vi "UDP_comm_state_machine.vi"(6 "Data to send":T1, 8 "error in (no error)":errorcluster, 9 "UDP State":T4, 11 "UDP Pproperties":T3={"Remote Host Port"=9999, "Remote Host IP"="127.0.0.1", "write_ID"=enum."0"}) -> (0 "error out":errorcluster, 1 "error code":i32, 3 "Data to read OUT":T2)   [LabVIEW 2012]
uses:
  UDP_state.ctl
  DataToSend.ctl
panel:
  out "error IO":errorcluster
  out "offset past number":i32
  out "substring":string
  out "number":dbl
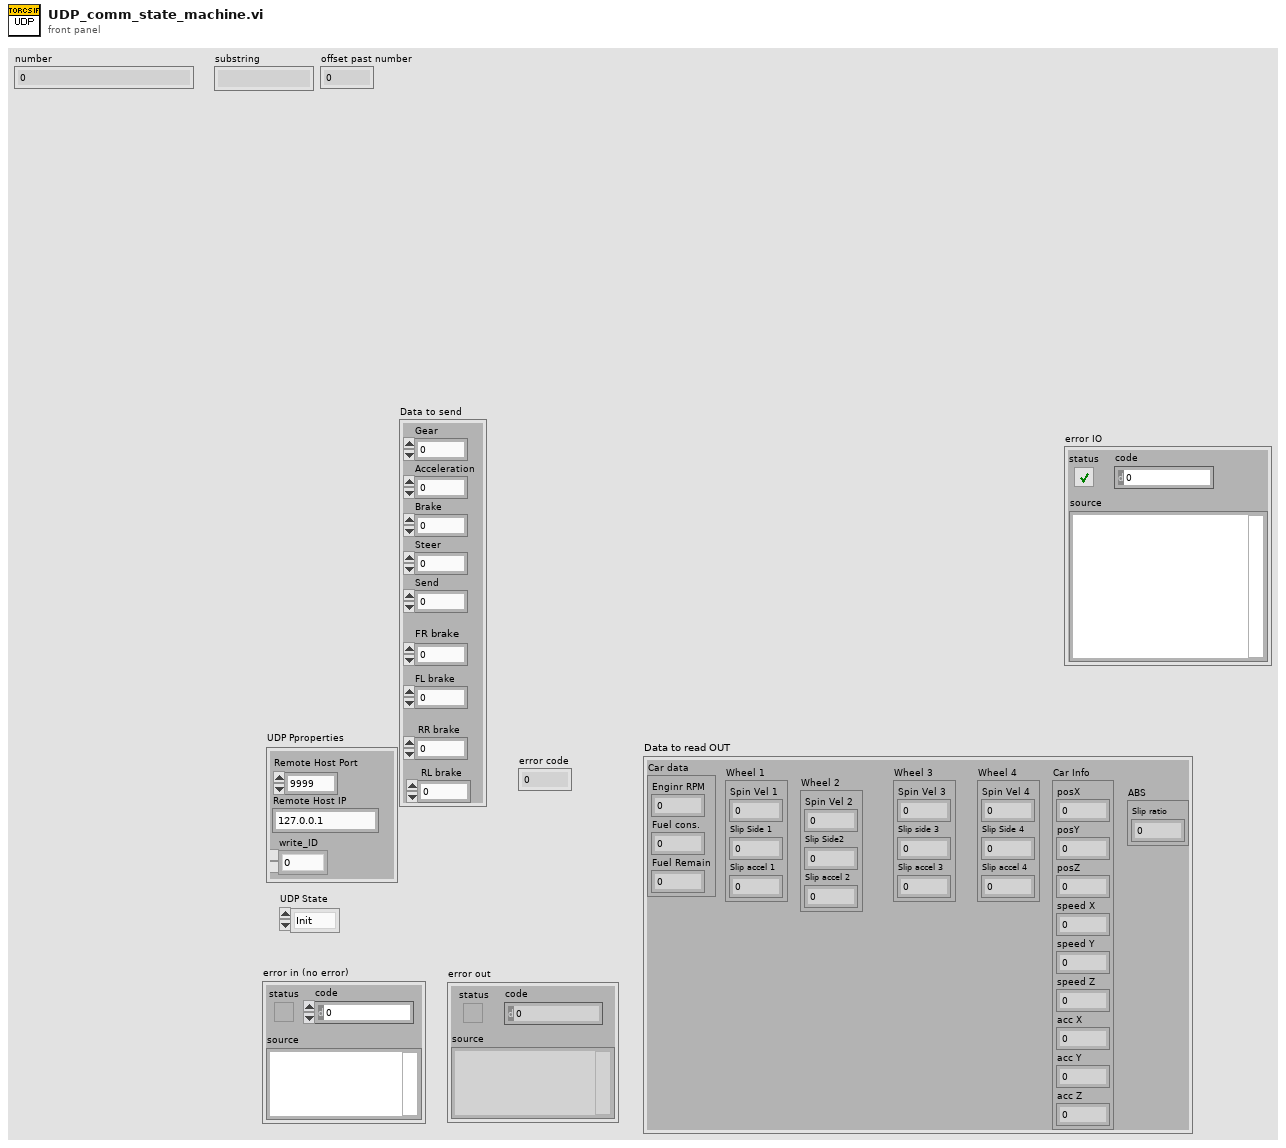
[diagram p1: front panel]
types:
  T1 = typedef "DataToSend.ctl" = cluster{"Gear":dbl, "Acceleration":dbl, "Brake":dbl, "Steer":dbl, "Send":dbl, "FR brake":dbl, "FL brake":dbl, " RR brake":dbl, " RL brake":dbl}
  T2 = cluster{"Car data ":cluster{"Enginr RPM":dbl, "Fuel cons.":dbl, "Fuel Remain":dbl}, "Wheel 1":cluster{"Spin Vel 1":dbl, "Slip Side 1":dbl, "Slip accel 1":dbl}, "Wheel 2":cluster{"Spin Vel 2":dbl, "Slip Side2":dbl, "Slip accel 2":dbl}, "Wheel 3":cluster{"Spin Vel 3":dbl, "Slip side 3":dbl, "Slip accel 3":dbl}, "Wheel 4":cluster{"Spin Vel 4":dbl, "Slip Side 4":dbl, "Slip accel 4":dbl}, "Car Info":cluster{"posX":dbl, "posY":dbl, "posZ":dbl, "speed X":dbl, "speed Y":dbl, "speed Z":dbl, "acc X":dbl, "acc Y":dbl, "acc Z":dbl}, "ABS":cluster{"Slip ratio":dbl}}
  T3 = cluster{"Remote Host Port":u16, "Remote Host IP":string, "write_ID":enum32{"0", "1", "2", "3", "4"}}
  T4 = typedef "UDP_state.ctl" = enum16{"Init", "Write", "Read", "Close"}
  T5 = cluster{"Enginr RPM":dbl, "Fuel cons.":dbl, "Fuel Remain":dbl}
  T6 = cluster{"posX":dbl, "posY":dbl, "posZ":dbl, "speed X":dbl, "speed Y":dbl, "speed Z":dbl, "acc X":dbl, "acc Y":dbl, "acc Z":dbl}
  T7 = cluster{"Spin Vel 1":dbl, "Slip Side 1":dbl, "Slip accel 1":dbl}
  T8 = cluster{"Spin Vel 2":dbl, "Slip Side2":dbl, "Slip accel 2":dbl}
  T9 = cluster{"Spin Vel 3":dbl, "Slip side 3":dbl, "Slip accel 3":dbl}
  T10 = cluster{"Spin Vel 4":dbl, "Slip Side 4":dbl, "Slip accel 4":dbl}
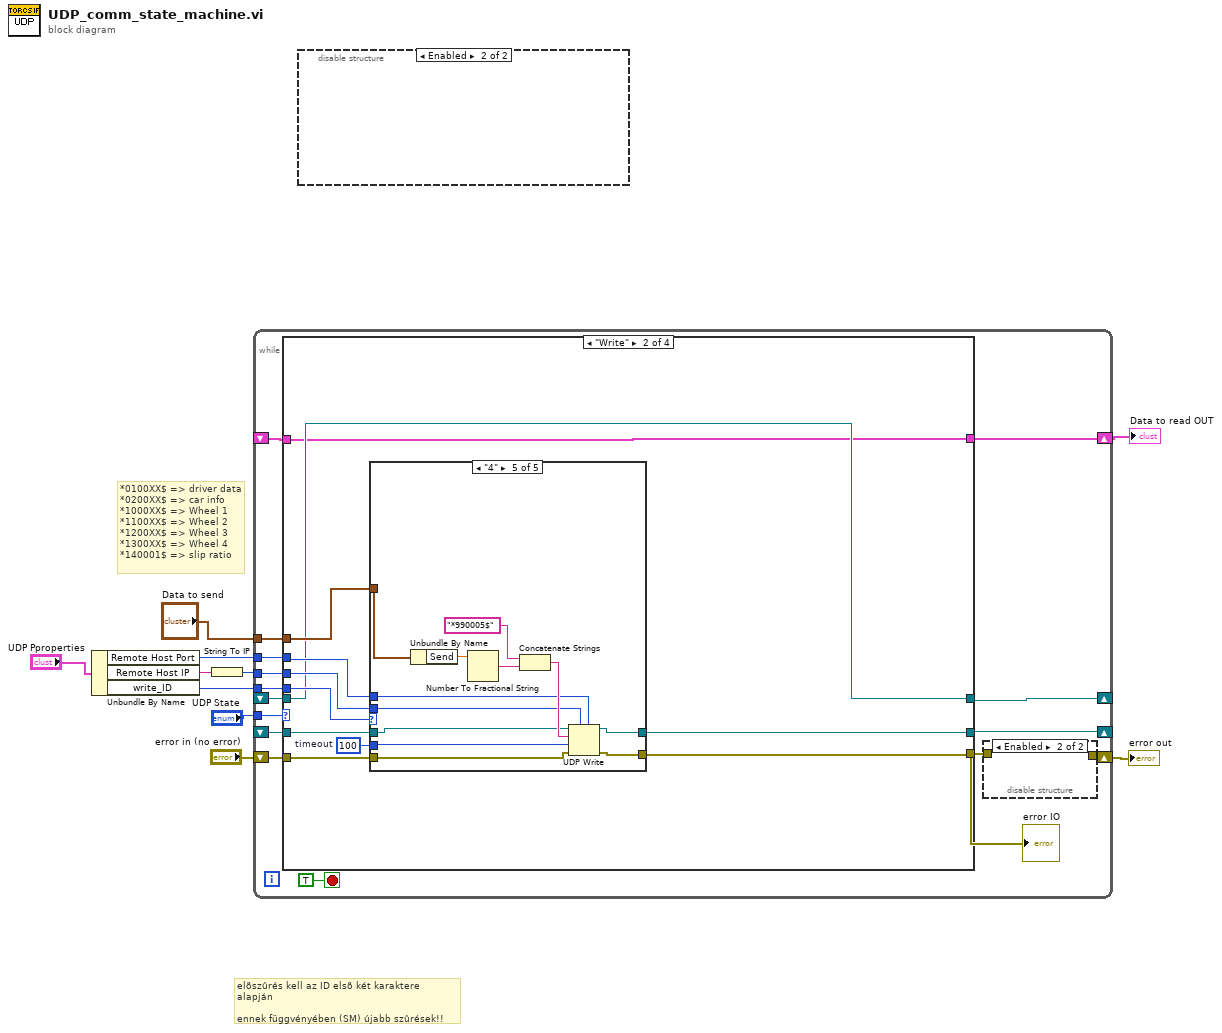
[diagram p0: block diagram]
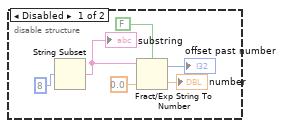
[diagram p2: hidden frame]
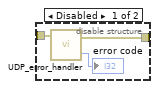
[diagram p3: hidden frame]
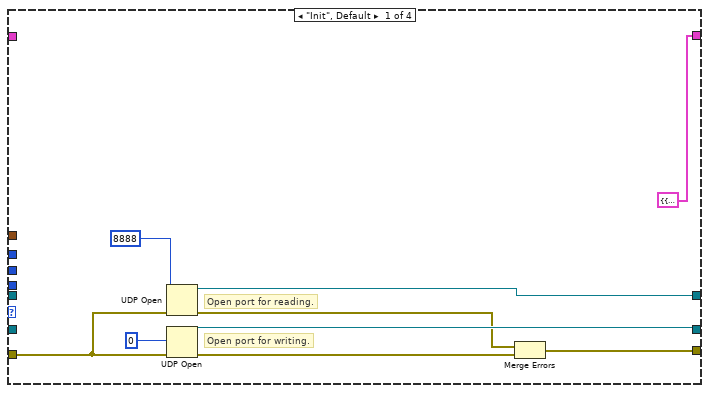
[diagram p4: hidden frame]
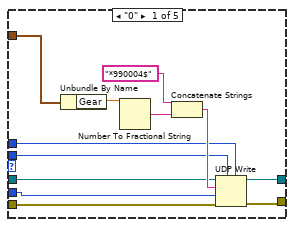
[diagram p5: hidden frame]
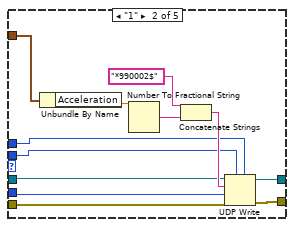
[diagram p6: hidden frame]
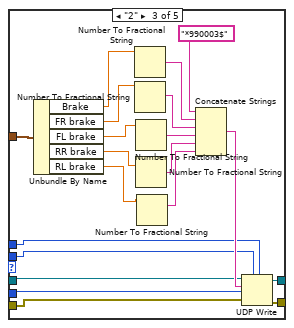
[diagram p7: hidden frame]
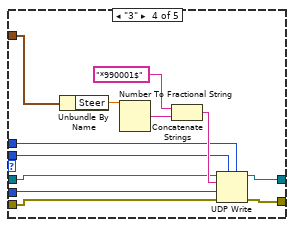
[diagram p8: hidden frame]
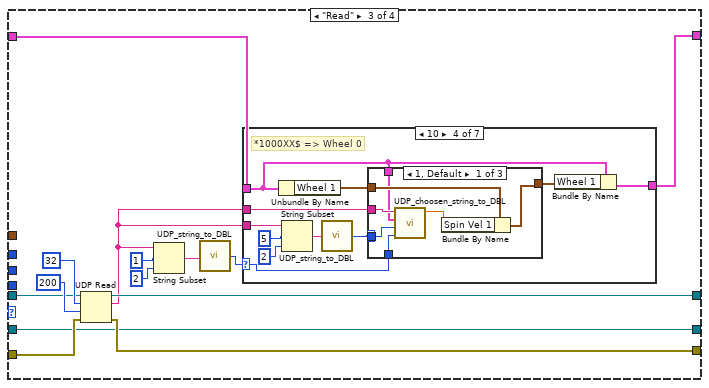
[diagram p9: hidden frame]
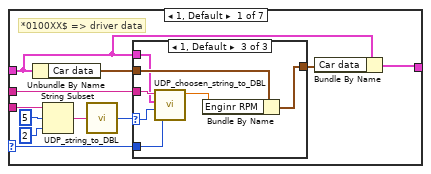
[diagram p10: hidden frame]
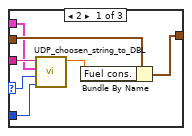
[diagram p11: hidden frame]
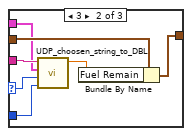
[diagram p12: hidden frame]
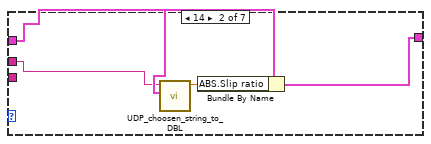
[diagram p13: hidden frame]
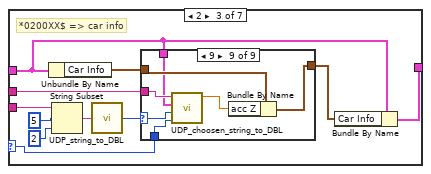
[diagram p14: hidden frame]
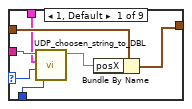
[diagram p15: hidden frame]
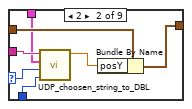
[diagram p16: hidden frame]
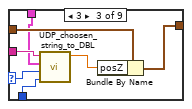
[diagram p17: hidden frame]
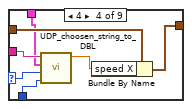
[diagram p18: hidden frame]
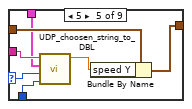
[diagram p19: hidden frame]
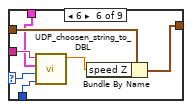
[diagram p20: hidden frame]
diagram:
  # "elõszûrés kell az ID elsõ két karaktere alapján\n\nennek függvényében (SM) újabb szûrések!!"
  # "*0100XX$ => driver data\n*0200XX$ => car info\n*1000XX$ => Wheel 1\n*1100XX$ => Wheel 2\n*1200XX$ => Wheel 3\n*1300XX$ => Wheel 4\n*140001$ => slip ratio"
  n1 = Unbundle By Name("UDP Pproperties") -> ("Remote Host Port"=w5:u16, "Remote Host IP"=w4:string, "write_ID"=w3:enum32{"0", "1", "2", "3", "4"})
  n2 = String To IP(1:w4) -> (0:w9:u32)
  n3 = while {
    shift-right: [w24] -> _
    shift-left: _ -> [w23]
    shift-right: [w13] -> w10
    shift-left: "error in (no error)" -> [w21]
    tunnel: "Data to send" -> [w22]
    shift-right: [w12] -> w2
    shift-left: _ -> [w11]
    tunnel: w5 -> [w20]
    tunnel: w9 -> [w19]
    tunnel: "UDP State" -> [w18]
    tunnel: w3 -> [w17]
    shift-right: [w16] -> _
    shift-left: _ -> [w15]
    stop <- TRUE stop-if-true
    n4 = case shown="\"Write\"" w18 {
      tunnel: [w37 w43 w124 w376] -> w24
      tunnel: w21 -> [w33 w47 w129 w374]
      tunnel: [w35 w42 w127 w372] -> w14
      tunnel: w23 -> [_ w48 w124 w377]
      tunnel: w22 -> [_ w46 _ _]
      tunnel: w11 -> [_ w39 w118 w369]
      tunnel: w20 -> [_ w45 _ _]
      tunnel: w19 -> [_ w44 _ _]
      tunnel: w17 -> [_ w41 _ _]
      tunnel: [w31 w40 w125 w370] -> w16
      tunnel: w15 -> [_ w40 w126 w375]
      tunnel: [T2 {"Car data "={"Enginr RPM"=0.0, "Fuel cons."=0.0, "Fuel Remain"=0.0}, "Wheel 1"={"Spin Vel 1"=0.0, "Slip Side 1"=0.0, "Slip accel 1"=0.0}, "Wheel 2"={"Spin Vel 2"=0.0, "Slip Side2"=0.0, "Slip accel 2"=0.0}, "Wheel 3"={"Spin Vel 3"=0.0, "Slip side 3"=0.0, "Slip accel 3"=0.0}, "Wheel 4"={"Spin Vel 4"=0.0, "Slip Side 4"=0.0, "Slip accel 4"=0.0}, "Car Info"={"posX"=0.0, "posY"=0.0, "posZ"=0.0, "speed X"=0.0, "speed Y"=0.0, "speed Z"=0.0, "acc X"=0.0, "acc Y"=0.0, "acc Z"=0.0}, "ABS"={"Slip ratio"=0.0}} ("Data to read OUT") w39 w119 w369] -> w12
      frame "Init", Default {
        # "Open port for writing."
        # "Open port for reading."
        n5 = UDP Open(8:w33, 11:u16 8888 ("port")) -> (port=w31:refnum<k16>, 0:w32:errorcluster)  [unwired: 3 in, 1 out]
        n6 = UDP Open(8:w33, 11:u16 0 ("port")) -> (port=w37:refnum<k16>, 0:w36:errorcluster)  [unwired: 3 in, 1 out]
        n7 = Merge Errors(w32, w36) -> (w35:errorcluster)
      }
      frame "Write" {
        w38 = 100  # timeout
        n8 = case shown="\"4\"" w41 {
          tunnel: w48 -> [w56 w63 w84 w97 w111]
          tunnel: w47 -> [w55 w61 w82 w96 w109]
          tunnel: w46 -> [w54 w66 w81 w100 w113]
          tunnel: w45 -> [w53 w65 w86 w98 w106]
          tunnel: w44 -> [w52 w64 w85 w99 w105]
          tunnel: [w51 w68 w87 w94 w107] -> w43
          tunnel: [w50 w67 w88 w93 w108] -> w42
          tunnel: w38 -> [w49 w62 w83 w95 w110]
          frame "0" {
            n9 = Unbundle By Name(w54) -> ("Gear"=w60:dbl)
            n10 = Number To Fractional String(number=w60) -> (F-format string=w59:string)  [unwired: 3 in]
            n11 = Concatenate Strings("*990004$", w59) -> (w58:string)
            n12 = UDP Write(address=w52, port or service name=w53, connection ID=w56, data in=w58, 8:w55, 9:w49) -> (error out=w50:errorcluster, 3:w51:refnum<k16>)
          }
          frame "1" {
            n13 = Unbundle By Name(w66) -> ("Acceleration"=w72:dbl)
            n14 = Number To Fractional String(number=w72) -> (F-format string=w71:string)  [unwired: 3 in]
            n15 = Concatenate Strings("*990002$", w71) -> (w69:string)
            n16 = UDP Write(address=w64, port or service name=w65, connection ID=w63, data in=w69, 8:w61, 9:w62) -> (error out=w67:errorcluster, 3:w68:refnum<k16>)
          }
          frame "2" {
            n17 = Unbundle By Name(w81) -> ("Brake"=w89:dbl, "FR brake"=w80:dbl, "FL brake"=w79:dbl, "RR brake"=w78:dbl, "RL brake"=w77:dbl)
            n18 = Number To Fractional String(number=w89) -> (F-format string=w91:string)  [unwired: 3 in]
            n19 = Number To Fractional String(number=w80) -> (F-format string=w76:string)  [unwired: 3 in]
            n20 = Number To Fractional String(number=w79) -> (F-format string=w75:string)  [unwired: 3 in]
            n21 = Number To Fractional String(number=w78) -> (F-format string=w74:string)  [unwired: 3 in]
            n22 = Number To Fractional String(number=w77) -> (F-format string=w73:string)  [unwired: 3 in]
            n23 = Concatenate Strings("*990003$", w91, w76, w75, w74, w73) -> (w92:string)
            n24 = UDP Write(address=w85, port or service name=w86, connection ID=w84, data in=w92, 8:w82, 9:w83) -> (error out=w88:errorcluster, 3:w87:refnum<k16>)
          }
          frame "3" {
            n25 = Unbundle By Name(w100) -> ("Steer"=w101:dbl)
            n26 = Number To Fractional String(number=w101) -> (F-format string=w103:string)  [unwired: 3 in]
            n27 = Concatenate Strings("*990001$", w103) -> (w102:string)
            n28 = UDP Write(address=w99, port or service name=w98, connection ID=w97, data in=w102, 8:w96, 9:w95) -> (error out=w93:errorcluster, 3:w94:refnum<k16>)
          }
          frame "4" {
            n29 = Unbundle By Name(w113) -> ("Send"=w112:dbl)
            n30 = Number To Fractional String(number=w112) -> (F-format string=w115:string)  [unwired: 3 in]
            n31 = Concatenate Strings("*990005$", w115) -> (w116:string)
            n32 = UDP Write(address=w105, port or service name=w106, connection ID=w111, data in=w116, 8:w109, 9:w110) -> (error out=w108:errorcluster, 3:w107:refnum<k16>)
          }
        }
      }
      frame "Read" {
        n33 = UDP Read(connection ID=w126, max size (548)=32, timeout ms (25000)=200, 8:w129) -> (data out=w117:string, error out=w127:errorcluster, 3:w125:refnum<k16>)  [unwired: 2 out]
        n34 = String Subset(string=w117, offset (0)=1, length (rest)=2 ("length (rest)")) -> (substring=w121:string)
        n35 = call "UDP_string_to_DBL.vi"("input string"=w121) -> ("output number"=w120:i32)
        n36 = case shown="10" w120 {
          selector: w120 -> [w133 _ w168 w243 w275 w308 w338]
          tunnel: w118 -> [w131 w165 w167 w242 w276 w305 w337]
          tunnel: w117 -> [w139 _ w170 w248 w280 w312 w344]
          tunnel: w117 -> [w137 w164 w171 w246 w274 w306 w340]
          tunnel: [w132 w166 w172 w244 w279 w311 w343] -> w119
          frame 1, Default {
            # "*0100XX$ => driver data"
            n37 = Unbundle By Name(w131) -> ("Car data"=w138:T5)
            n38 = String Subset(string=w139, offset (0)=5, length (rest)=2 ("length (rest)")) -> (substring=w136:string)
            n39 = call "UDP_string_to_DBL.vi"("input string"=w136) -> ("output number"=w134:i32)
            n40 = case shown="1, Default" w134 {
              selector: w134 -> [w144 w151 w158]
              tunnel: w138 -> [w147 w154 w162]
              tunnel: w137 -> [w145 w152 w159]
              tunnel: [w146 w153 w160] -> w135
              tunnel: w133 -> [w143 w150 w157]
              tunnel: w131 -> [w142 w149 w156]
              frame 2 {
                n41 = call "UDP_choosen_string_to_DBL.vi"("main ID"=w143, "secondary ID"=w144, "Data to read"=w142, "input string"=w145) -> ("output number"=w148:dbl)  [unwired: 3 in]
                n42 = Bundle By Name(cluster=w147, "Fuel cons."=w148) -> (w146:T5)
              }
              frame 3 {
                n43 = call "UDP_choosen_string_to_DBL.vi"("main ID"=w150, "secondary ID"=w151, "Data to read"=w149, "input string"=w152) -> ("output number"=w155:dbl)  [unwired: 3 in]
                n44 = Bundle By Name(cluster=w154, "Fuel Remain"=w155) -> (w153:T5)
              }
              frame 1, Default {
                n45 = call "UDP_choosen_string_to_DBL.vi"("main ID"=w157, "secondary ID"=w158, "Data to read"=w156, "input string"=w159) -> ("output number"=w161:dbl)  [unwired: 3 in]
                n46 = Bundle By Name(cluster=w162, "Enginr RPM"=w161) -> (w160:T5)
              }
            }
            n47 = Bundle By Name(cluster=w131, "Car data"=w135) -> (w132:T2)
          }
          frame 14 {
            n48 = call "UDP_choosen_string_to_DBL.vi"("Data to read"=w165, "input string"=w164) -> ("output number"=w163:dbl)  [unwired: 5 in]
            n49 = Bundle By Name(cluster=w165, "ABS.Slip ratio"=w163) -> (w166:T2)
          }
          frame 2 {
            # "*0200XX$ => car info"
            n50 = Unbundle By Name(w167) -> ("Car Info"=w174:T6)
            n51 = String Subset(string=w170, offset (0)=5, length (rest)=2 ("length (rest)")) -> (substring=w175:string)
            n52 = call "UDP_string_to_DBL.vi"("input string"=w175) -> ("output number"=w169:i32)
            n53 = case shown="9" w169 {
              selector: w169 -> [w180 w186 w193 w200 w207 w215 w222 w228 w236]
              tunnel: w174 -> [w184 w188 w196 w204 w211 w217 w225 w231 w238]
              tunnel: w171 -> [w181 w190 w195 w203 w210 w216 w224 w232 w239]
              tunnel: [w182 w189 w197 w202 w209 w218 w223 w230 w237] -> w173
              tunnel: w168 -> [w179 w185 w192 w199 w206 w214 w221 w229 w235]
              tunnel: w167 -> [w178 w187 w194 w201 w208 w213 w220 w227 w234]
              frame 1, Default {
                n54 = call "UDP_choosen_string_to_DBL.vi"("main ID"=w179, "secondary ID"=w180, "Data to read"=w178, "input string"=w181) -> ("output number"=w183:dbl)  [unwired: 3 in]
                n55 = Bundle By Name(cluster=w184, "posX"=w183) -> (w182:T6)
              }
              frame 2 {
                n56 = call "UDP_choosen_string_to_DBL.vi"("main ID"=w185, "secondary ID"=w186, "Data to read"=w187, "input string"=w190) -> ("output number"=w191:dbl)  [unwired: 3 in]
                n57 = Bundle By Name(cluster=w188, "posY"=w191) -> (w189:T6)
              }
              frame 3 {
                n58 = call "UDP_choosen_string_to_DBL.vi"("main ID"=w192, "secondary ID"=w193, "Data to read"=w194, "input string"=w195) -> ("output number"=w198:dbl)  [unwired: 3 in]
                n59 = Bundle By Name(cluster=w196, "posZ"=w198) -> (w197:T6)
              }
              frame 4 {
                n60 = call "UDP_choosen_string_to_DBL.vi"("main ID"=w199, "secondary ID"=w200, "Data to read"=w201, "input string"=w203) -> ("output number"=w205:dbl)  [unwired: 3 in]
                n61 = Bundle By Name(cluster=w204, "speed X"=w205) -> (w202:T6)
              }
              frame 5 {
                n62 = call "UDP_choosen_string_to_DBL.vi"("main ID"=w206, "secondary ID"=w207, "Data to read"=w208, "input string"=w210) -> ("output number"=w212:dbl)  [unwired: 3 in]
                n63 = Bundle By Name(cluster=w211, "speed Y"=w212) -> (w209:T6)
              }
              frame 6 {
                n64 = call "UDP_choosen_string_to_DBL.vi"("main ID"=w214, "secondary ID"=w215, "Data to read"=w213, "input string"=w216) -> ("output number"=w219:dbl)  [unwired: 3 in]
                n65 = Bundle By Name(cluster=w217, "speed Z"=w219) -> (w218:T6)
              }
              frame 7 {
                n66 = call "UDP_choosen_string_to_DBL.vi"("main ID"=w221, "secondary ID"=w222, "Data to read"=w220, "input string"=w224) -> ("output number"=w226:dbl)  [unwired: 3 in]
                n67 = Bundle By Name(cluster=w225, "acc X"=w226) -> (w223:T6)
              }
              frame 8 {
                n68 = call "UDP_choosen_string_to_DBL.vi"("main ID"=w229, "secondary ID"=w228, "Data to read"=w227, "input string"=w232) -> ("output number"=w233:dbl)  [unwired: 3 in]
                n69 = Bundle By Name(cluster=w231, "acc Y"=w233) -> (w230:T6)
              }
              frame 9 {
                n70 = call "UDP_choosen_string_to_DBL.vi"("main ID"=w235, "secondary ID"=w236, "Data to read"=w234, "input string"=w239) -> ("output number"=w240:dbl)  [unwired: 3 in]
                n71 = Bundle By Name(cluster=w238, "acc Z"=w240) -> (w237:T6)
              }
            }
            n72 = Bundle By Name(cluster=w167, "Car Info"=w173) -> (w172:T2)
          }
          frame 10 {
            # "*1000XX$ => Wheel 0"
            n73 = Unbundle By Name(w242) -> ("Wheel 1"=w247:T7)
            n74 = String Subset(string=w248, offset (0)=5, length (rest)=2 ("length (rest)")) -> (substring=w249:string)
            n75 = call "UDP_string_to_DBL.vi"("input string"=w249) -> ("output number"=w241:i32)
            n76 = case shown="1, Default" w241 {
              selector: w241 -> [w254 w260 w267]
              tunnel: w247 -> [w258 w262 w270]
              tunnel: w246 -> [w255 w264 w269]
              tunnel: [w256 w263 w271] -> w245
              tunnel: w243 -> [w253 w259 w266]
              tunnel: w242 -> [w252 w261 w268]
              tunnel: w241 -> [_ _ _]
              frame 1, Default {
                n77 = call "UDP_choosen_string_to_DBL.vi"("main ID"=w253, "secondary ID"=w254, "Data to read"=w252, "input string"=w255) -> ("output number"=w257:dbl)  [unwired: 3 in]
                n78 = Bundle By Name(cluster=w258, "Spin Vel 1"=w257) -> (w256:T7)
              }
              frame 2 {
                n79 = call "UDP_choosen_string_to_DBL.vi"("main ID"=w259, "secondary ID"=w260, "Data to read"=w261, "input string"=w264) -> ("output number"=w265:dbl)  [unwired: 3 in]
                n80 = Bundle By Name(cluster=w262, "Slip Side 1"=w265) -> (w263:T7)
              }
              frame 3 {
                n81 = call "UDP_choosen_string_to_DBL.vi"("main ID"=w266, "secondary ID"=w267, "Data to read"=w268, "input string"=w269) -> ("output number"=w272:dbl)  [unwired: 3 in]
                n82 = Bundle By Name(cluster=w270, "Slip accel 1"=w272) -> (w271:T7)
              }
            }
            n83 = Bundle By Name(cluster=w242, "Wheel 1"=w245) -> (w244:T2)
          }
          frame 11 {
            # "*1100XX$ => Wheel 2"
            n84 = Unbundle By Name(w276) -> ("Wheel 2"=w278:T8)
            n85 = String Subset(string=w280, offset (0)=5, length (rest)=2 ("length (rest)")) -> (substring=w281:string)
            n86 = call "UDP_string_to_DBL.vi"("input string"=w281) -> ("output number"=w273:i32)
            n87 = case shown="3" w273 {
              selector: w273 -> [w287 w292 w299]
              tunnel: w278 -> [w290 w294 w302]
              tunnel: w274 -> [w284 w296 w301]
              tunnel: [w288 w295 w303] -> w277
              tunnel: w275 -> [w286 w291 w298]
              tunnel: w276 -> [w285 w293 w300]
              frame 1, Default {
                n88 = call "UDP_choosen_string_to_DBL.vi"("main ID"=w286, "secondary ID"=w287, "Data to read"=w285, "input string"=w284) -> ("output number"=w289:dbl)  [unwired: 3 in]
                n89 = Bundle By Name(cluster=w290, "Spin Vel 2"=w289) -> (w288:T8)
              }
              frame 2 {
                n90 = call "UDP_choosen_string_to_DBL.vi"("main ID"=w291, "secondary ID"=w292, "Data to read"=w293, "input string"=w296) -> ("output number"=w297:dbl)  [unwired: 3 in]
                n91 = Bundle By Name(cluster=w294, "Slip Side2"=w297) -> (w295:T8)
              }
              frame 3 {
                n92 = call "UDP_choosen_string_to_DBL.vi"("main ID"=w298, "secondary ID"=w299, "Data to read"=w300, "input string"=w301) -> ("output number"=w304:dbl)  [unwired: 3 in]
                n93 = Bundle By Name(cluster=w302, "Slip accel 2"=w304) -> (w303:T8)
              }
            }
            n94 = Bundle By Name(cluster=w276, "Wheel 2"=w277) -> (w279:T2)
          }
          frame 12 {
            # "*1200XX$ => Wheel 3"
            n95 = Unbundle By Name(w305) -> ("Wheel 3"=w310:T9)
            n96 = String Subset(string=w312, offset (0)=5, length (rest)=2 ("length (rest)")) -> (substring=w313:string)
            n97 = call "UDP_string_to_DBL.vi"("input string"=w313) -> ("output number"=w307:i32)
            n98 = case shown="1, Default" w307 {
              selector: w307 -> [w319 w324 w331]
              tunnel: w310 -> [w322 w326 w334]
              tunnel: w306 -> [w316 w328 w333]
              tunnel: [w320 w327 w335] -> w309
              tunnel: w308 -> [w318 w323 w330]
              tunnel: w305 -> [w317 w325 w332]
              frame 1, Default {
                n99 = call "UDP_choosen_string_to_DBL.vi"("main ID"=w318, "secondary ID"=w319, "Data to read"=w317, "input string"=w316) -> ("output number"=w321:dbl)  [unwired: 3 in]
                n100 = Bundle By Name(cluster=w322, "Spin Vel 3"=w321) -> (w320:T9)
              }
              frame 2 {
                n101 = call "UDP_choosen_string_to_DBL.vi"("main ID"=w323, "secondary ID"=w324, "Data to read"=w325, "input string"=w328) -> ("output number"=w329:dbl)  [unwired: 3 in]
                n102 = Bundle By Name(cluster=w326, "Slip side 3"=w329) -> (w327:T9)
              }
              frame 3 {
                n103 = call "UDP_choosen_string_to_DBL.vi"("main ID"=w330, "secondary ID"=w331, "Data to read"=w332, "input string"=w333) -> ("output number"=w336:dbl)  [unwired: 3 in]
                n104 = Bundle By Name(cluster=w334, "Slip accel 3"=w336) -> (w335:T9)
              }
            }
            n105 = Bundle By Name(cluster=w305, "Wheel 3"=w309) -> (w311:T2)
          }
          frame 13 {
            # "*1300XX$ => Wheel 4"
            n106 = Unbundle By Name(w337) -> ("Wheel 4"=w341:T10)
            n107 = String Subset(string=w344, offset (0)=5, length (rest)=2 ("length (rest)")) -> (substring=w345:string)
            n108 = call "UDP_string_to_DBL.vi"("input string"=w345) -> ("output number"=w339:i32)
            n109 = case shown="1, Default" w339 {
              selector: w339 -> [w351 w356 w363]
              tunnel: w341 -> [w354 w358 w366]
              tunnel: w340 -> [w348 w360 w365]
              tunnel: [w352 w359 w367] -> w342
              tunnel: w338 -> [w350 w355 w362]
              tunnel: w337 -> [w349 w357 w364]
              frame 1, Default {
                n110 = call "UDP_choosen_string_to_DBL.vi"("main ID"=w350, "secondary ID"=w351, "Data to read"=w349, "input string"=w348) -> ("output number"=w353:dbl)  [unwired: 3 in]
                n111 = Bundle By Name(cluster=w354, "Spin Vel 4"=w353) -> (w352:T10)
              }
              frame 2 {
                n112 = call "UDP_choosen_string_to_DBL.vi"("main ID"=w355, "secondary ID"=w356, "Data to read"=w357, "input string"=w360) -> ("output number"=w361:dbl)  [unwired: 3 in]
                n113 = Bundle By Name(cluster=w358, "Slip Side 4"=w361) -> (w359:T10)
              }
              frame 3 {
                n114 = call "UDP_choosen_string_to_DBL.vi"("main ID"=w362, "secondary ID"=w363, "Data to read"=w364, "input string"=w365) -> ("output number"=w368:dbl)  [unwired: 3 in]
                n115 = Bundle By Name(cluster=w366, "Slip accel 4"=w368) -> (w367:T10)
              }
            }
            n116 = Bundle By Name(cluster=w337, "Wheel 4"=w342) -> (w343:T2)
          }
        }
      }
      frame "Close" {
        n117 = UDP Close(connection ID=w375, 8:w374) -> (connection ID out=w370:refnum<k16>, error out=w371:errorcluster)
        n118 = UDP Close(connection ID=w377, 8:w374) -> (connection ID out=w376:refnum<k16>, error out=w373:errorcluster)
        n119 = Merge Errors(w371, w373) -> (w372:errorcluster)
      }
    }
    "error IO" <- w14
    n120 = disable-structure shown="Enabled" {
      disable-tunnel: w14 -> [w28 _]
      disable-tunnel: [w27 _] -> w13
      frame Disabled {
        n121 = call "UDP_error_handler.vi"("error in (no error)"=w28) -> ("error out"=w27:errorcluster, "error code"=→"error code":i32)
      }
      frame Enabled {
      }
    }
  }
  "error out" <- w10
  "Data to read OUT" <- w2
  n122 = disable-structure shown="Enabled" {
    frame Disabled {
      n123 = String Subset(offset (0)=8 ("offset")) -> (string=w382:string, substring=w384:string)  [unwired: 1 in]
      "substring" <- w384
      n124 = Fract/Exp String To Number(use system decimal point (T)=FALSE, string=w384, default (0 dbl)=0.0 ("default (0 DBL)")) -> (offset past number=→"offset past number":i32, number=→"number":dbl)  [unwired: 1 in]
    }
    frame Enabled {
    }
  }
